vi "New_Data.vi"(8 "error in":errorcluster, 10 "Graph_Data":T1 {"ЦАП, градС" format="%.3g"; "Тнагр, градС" format="%.3g"; "Q, мл" format="%.3g"; "Рдм, МПа" format="%.3g"; "Vпл, см3" format="Р2 %#.2f МПа"; "Рэфф, МПа" format="%.3g"; "dL, мм" format="%.4f"; "R, Ом" format="%.4f"; "Ргор, МПа" format="%.2f град.С"; "Рпл2, МПа" format="Р2 %#.2f МПа"; "Рпл1, МПа" format="Р2 %#.2f МПа"}) -> (0 "error out":errorcluster)   [LabVIEW 2023, in "Graph_data_collector.lvlib"]
doc: "_____\nCreated using DQMH Event Scripter 6.1.0.128."
uses:
  Graph_data_collector.lvlib
  Data Control.ctl
  New_Data Argument--cluster.ctl
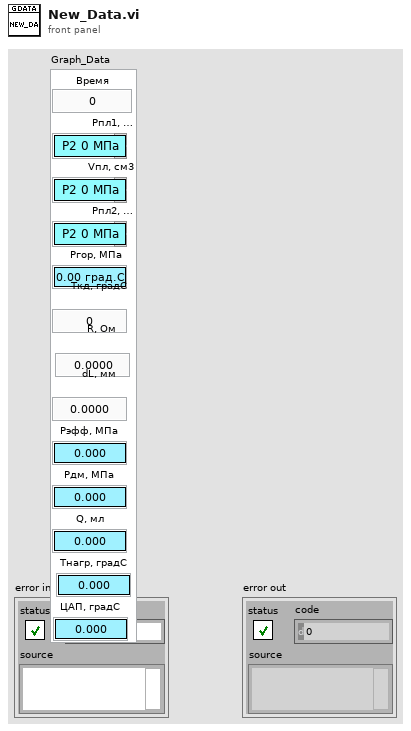
[diagram p1: front panel]
types:
  T1 = typedef "Graph_data_collector.lvlib/Data Control.ctl" = cluster{"Время":dbl, "Рпл1, МПа":dbl, "Vпл, см3":dbl, "Рпл2, МПа":dbl, "Ргор, МПа":dbl, "Ткд, градС":dbl, "R, Ом":dbl, "dL, мм":dbl, "Рэфф, МПа":dbl, "Рдм, МПа":dbl, "Q, мл":dbl, "Тнагр, градС":dbl, "ЦАП, градС":dbl}
  T2 = typedef "Graph_data_collector.lvlib/New_Data Argument--cluster.ctl" = cluster{"Graph_Data":T1}
  T3 = typedef "Graph_data_collector.lvlib/Request Events--cluster.ctl" = cluster{"Stop Module":refnum<user-event>, "Show Panel":refnum<user-event>, "Hide Panel":refnum<user-event>, "Get Module Execution Status":refnum<user-event>, "Show Diagram":refnum<user-event>, "New_Data":refnum<user-event>}
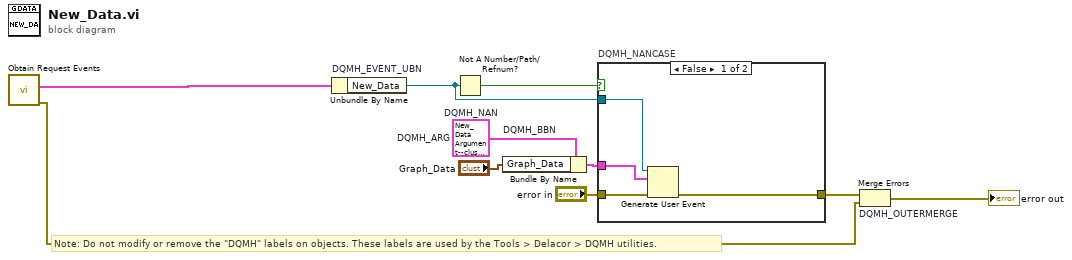
[diagram p0: block diagram]
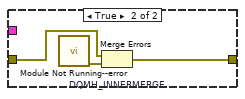
[diagram p2: hidden frame]
diagram:
  w4 = T2 {"Graph_Data"={"Время"=0.0, "Рпл1, МПа"=0.0, "Vпл, см3"=0.0, "Рпл2, МПа"=0.0, "Ргор, МПа"=0.0, "Ткд, градС"=0.0, "R, Ом"=0.0, "dL, мм"=0.0, "Рэфф, МПа"=0.0, "Рдм, МПа"=0.0, "Q, мл"=0.0, "Тнагр, градС"=0.0, "ЦАП, градС"=0.0}}  # DQMH_ARG
  # "Note: Do not modify or remove the \"DQMH\" labels on objects. These labels are used by the Tools > Delacor > DQMH utilities."
  n1 = call "Obtain Request Events.vi"() -> ("error out"=w2:errorcluster, "Graph_data_collector Request Events"=w1:T3)  [unwired: 10 in]
  n2 = Unbundle By Name "DQMH_EVENT_UBN"(w1) -> ("New_Data"=w6:refnum<user-event>)
  n3 = Not A Number/Path/Refnum? "DQMH_NAN"(number/path/refnum=w6) -> (NaN/Path/Refnum?=w7:bool)
  n4 = Bundle By Name "DQMH_BBN"(cluster=w4, "Graph_Data"="Graph_Data") -> (w8:T2)
  n5 = case "DQMH_NANCASE" shown="False" w7 {
    tunnel: "error in" -> [w14 w17]
    tunnel: [w13 w16] -> w5
    tunnel: w6 -> [w12 _]
    tunnel: w8 -> [w11 _]
    frame False {
      n6 = Generate User Event(user event=w12, event data cluster=w11, error in=w14) -> (error out=w13:errorcluster)  [unwired: 1 in, 1 out]
    }
    frame True {
      n7 = call "Module Not Running--error.vi"() -> ("error out"=w15:errorcluster)  [unwired: 11 in]
      n8 = Merge Errors "DQMH_INNERMERGE"(w17, w15) -> (w16:errorcluster)
    }
  }
  n9 = Merge Errors "DQMH_OUTERMERGE"(w5, w2) -> (→"error out":errorcluster)
